vi "DevB.Check Status.vi"(8 "error in (no error)":errorcluster, 11 "DevB Session in":T1) -> (0 "error out":errorcluster, 2 "Connected":bool, 3 "DevB Session out":T1)   [LabVIEW 2018]
uses:
  typedefs/DevB.Session.ctl
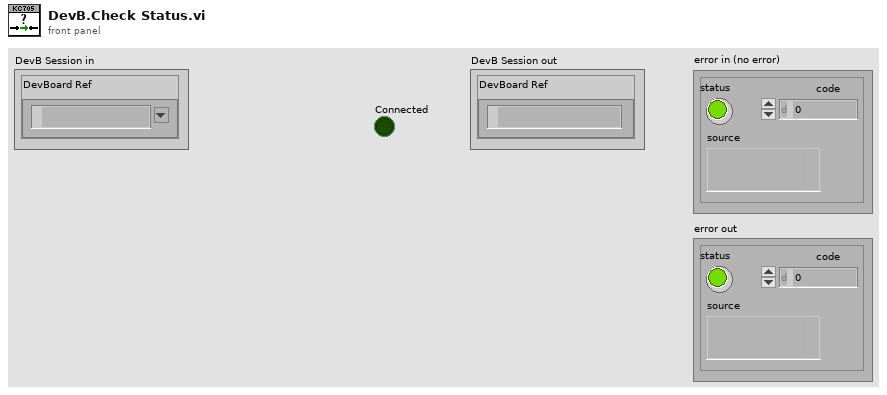
[diagram p1: front panel]
types:
  T1 = typedef "DevB.Session.ctl" = cluster{"DevBoard Ref":refnum<visa-resource-name>}
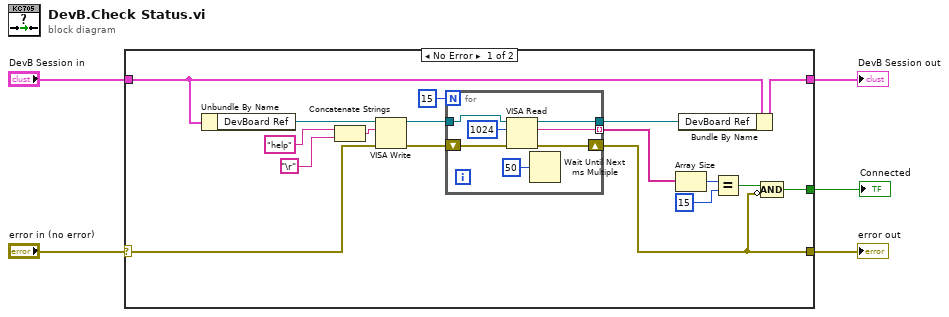
[diagram p0: block diagram]
diagram:
  n1 = case shown="No Error" "error in (no error)" {
    selector: "error in (no error)" -> [w20 w31]
    tunnel: "DevB Session in" -> [w21 w30]
    tunnel: [w6 w31] -> w3
    tunnel: [w19 w30] -> w2
    tunnel: [w7 _] -> w1
    frame No Error {
      n2 = Unbundle By Name(w21) -> ("DevBoard Ref"=w22:refnum<visa-resource-name>)
      n3 = Concatenate Strings("help" ("write buffer"), "\r") -> (w12:string)
      n4 = VISA Write(VISA resource name=w22, write buffer=w12, error in (no error)=w20) -> (VISA resource name out=w17:refnum<visa-resource-name>, error out=w15:errorcluster)  [unwired: 1 out]
      n5 = for {
        N: 15 -> [_]
        tunnel: [w24] -> w9 mode=indexing
        shift-right: [w26] -> w6
        shift-left: w15 -> [w27]
        tunnel: w17 -> [w29]
        tunnel: [w28] -> w16
        n6 = VISA Read(VISA resource name=w29, byte count=u32 1024, error in (no error)=w27) -> (VISA resource name out=w28:refnum<visa-resource-name>, read buffer=w24:string, error out=w26:errorcluster)  [unwired: 1 out]
        n7 = Wait Until Next ms Multiple(millisecond multiple=u32 50) -> ()  [unwired: 1 out]
      }
      n8 = Array Size(array=w9) -> (size(s)=w8:i32)
      n9 = Bundle By Name(cluster=w21, "DevBoard Ref"=w16) -> (w19:T1)
      n10 = Equal?(x=w8, y=15 ("x")) -> (x = y?=w14:bool)
      n11 = Compound Arithmetic op=AND(w14, invert w6) -> (w7:bool)
    }
    frame Error {
    }
  }
  "DevB Session out" <- w2
  "error out" <- w3
  "Connected" <- w1
